vi "CycleSelection_CycleSelected_Comparison.vi"(8 "Error In":errorcluster, 10 "Board Index":i32, 11 "GEA2 Reference In":refnum<k24>) -> (0 "Error Out":errorcluster, 1 "F09D Reading":string, 2 "200A Reading":string, 3 "GEA2 Reference Out":refnum<k24>, 4 "Pass/Fail?":bool)   [LabVIEW 2016]
uses:
  Q:/Common/DLLs/GEA3/GeaCommunication.dll
  Common/DLLs/GEA3/GeaCommunication.dll
  Common/LabVIEW GEA2 Toolkit/LabVIEW_GEA2_Toolkit.lvlibp/type defs/Source_Destination.ctl
  Common/LabVIEW GEA2 Toolkit/LabVIEW_GEA2_Toolkit.lvlibp/type defs/ERD Read Data In.ctl
  Common/LabVIEW GEA2 Toolkit/LabVIEW_GEA2_Toolkit.lvlibp/type defs/Data Type.ctl
  <vilib>/regexp/Match Regular Expression.xnode
  Common/LabVIEW GEA2 Toolkit/LabVIEW_GEA2_Toolkit.lvlibp
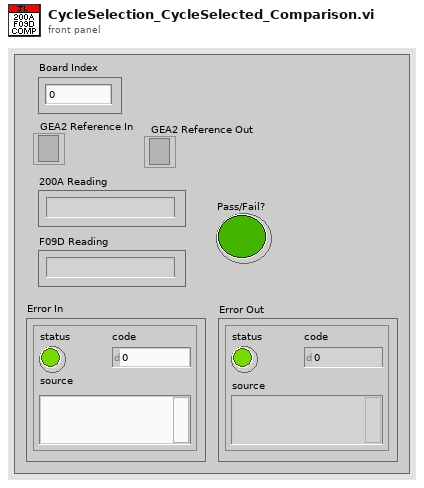
[diagram p1: front panel]
types:
  T1 = typedef "LabVIEW_GEA2_Toolkit.lvlibp/ERD Read Data In.ctl" = cluster{"ERD Number":u16, "Data Type":T2}
  T2 = typedef "LabVIEW_GEA2_Toolkit.lvlibp/Data Type.ctl" = enum16{"string", "boolean", "uint8_t", "uint16_t", "uint32_t", "uint64_t", "int8_t", "int16_t", "int32_t", "int64_t"}
  T3 = typedef "LabVIEW_GEA2_Toolkit.lvlibp/Source_Destination.ctl" = cluster{"Source":u8, "Destination":u8}
  T4 = typedef "LabVIEW_GEA2_Toolkit.lvlibp/ERD Read Data Out.ctl" = cluster{"ERD Number":u16, "Data":string}
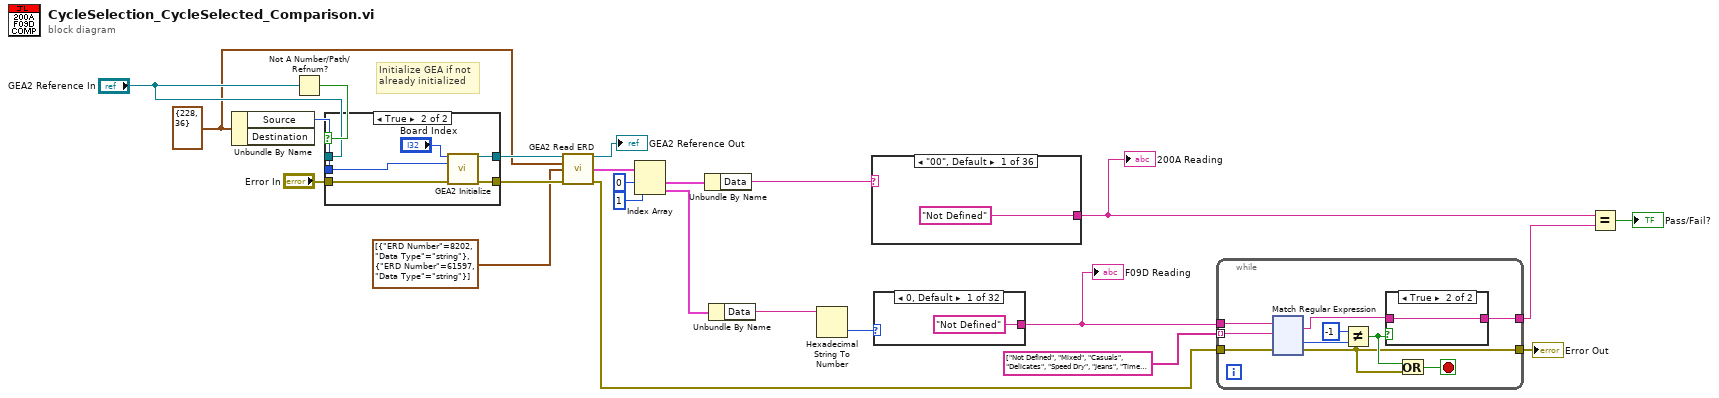
[diagram p0: block diagram]
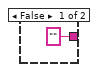
[diagram p2: hidden frame]
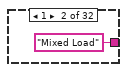
[diagram p3: hidden frame]
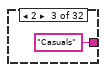
[diagram p4: hidden frame]
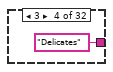
[diagram p5: hidden frame]
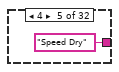
[diagram p6: hidden frame]
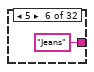
[diagram p7: hidden frame]
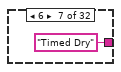
[diagram p8: hidden frame]
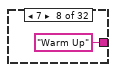
[diagram p9: hidden frame]
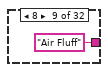
[diagram p10: hidden frame]
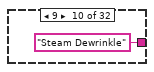
[diagram p11: hidden frame]
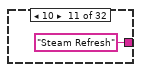
[diagram p12: hidden frame]
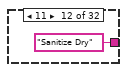
[diagram p13: hidden frame]
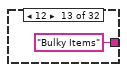
[diagram p14: hidden frame]
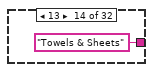
[diagram p15: hidden frame]
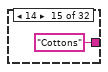
[diagram p16: hidden frame]
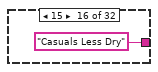
[diagram p17: hidden frame]
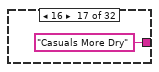
[diagram p18: hidden frame]
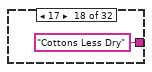
[diagram p19: hidden frame]
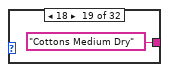
[diagram p20: hidden frame]
diagram:
  w13 = T3 {"Source"=228, "Destination"=36} ("GEA Inputs")
  # "Initialize GEA if not\nalready initialized"
  n1 = Unbundle By Name(w13) -> ("Source"=w23:u8)  [unwired: 1 out]
  n2 = Not A Number/Path/Refnum?(number/path/refnum="GEA2 Reference In") -> (NaN/Path/Refnum?=w24:bool)
  n3 = case shown="True" w24 {
    tunnel: "Error In" -> [w25 w31]
    tunnel: [w25 w30] -> w19
    tunnel: "GEA2 Reference In" -> [w26 _]
    tunnel: [w26 w29] -> w20
    tunnel: w23 -> [_ w28]
    frame False {
    }
    frame True {
      n4 = call "GEA2 Initialize.vi"("Board Index"="Board Index", "Source Address"=w28, "error in"=w31) -> ("GEA2 Reference Out"=w29:refnum<k24>, "error out"=w30:errorcluster)  [unwired: 10 in, 1 out]
    }
  }
  n5 = call "GEA2 Read ERD.vi"("GEA2 Reference In"=w20, "GEA Inputs"=w13, "Read ERD List"=T1[] [{"ERD Number"=8202, "Data Type"=enum."string"}, {"ERD Number"=61597, "Data Type"=enum."string"}], "Error In"=w19) -> ("GEA2 Reference Out"=→"GEA2 Reference Out":refnum<k24>, "ERD Data Out"=w18:T4[], "Error Out"=w6:errorcluster)  [unwired: 8 in, 1 out]
  n6 = Index Array(array=w18, index #1=0 ("index"), index #2=1 ("index")) -> (element #1=w16:T4, element #2=w10:T4)
  n7 = Unbundle By Name(w16) -> ("Data"=w15:string)
  n8 = Unbundle By Name(w10) -> ("Data"=w9:string)
  n9 = Hexadecimal String To Number(string=w9) -> (number=w14:u32)  [unwired: 2 in, 1 out]
  n10 = case shown="\"00\", Default" w15 {
    tunnel: ["Not Defined" "Basket Clean" "Drain & Spin" "Quick Rinse" "Bulky Items" "Sanitize" "Towels & Sheets" "Steam Refresh" "Normal/Mixed" "Whites" "Dark Colors" "Jeans" "Hand Wash" "Delicates" "Speed Wash" "Heavy Duty" "Allergen" "Power Clean" "Rinse & Spin" "Single Item" "Colors" "Cold Wash" "Cottons" "Easy Care" "Active Wear" "Timed Dry" "Dewrinkle" "Air Fluff" "Steam Refresh" "Steam Dewrinkle" "Speed Dry" "Mixed" "Quick Dry" "Casuals" "Warm Up" "Energy Saver"] -> w4
    frame "00", Default {
    }
    frame "01" {
    }
    frame "02" {
    }
    frame "03" {
    }
    frame "04" {
    }
    frame "05" {
    }
    frame "06" {
    }
    frame "07" {
    }
    frame "08" {
    }
    frame "09" {
    }
    frame "0A" {
    }
    frame "0B" {
    }
    frame "0C" {
    }
    frame "0D" {
    }
    frame "0E" {
    }
    frame "0F" {
    }
    frame "10" {
    }
    frame "11" {
    }
    frame "12" {
    }
    frame "13" {
    }
    frame "14" {
    }
    frame "15" {
    }
    frame "80" {
    }
    frame "81" {
    }
    frame "82" {
    }
    frame "83" {
    }
    frame "84" {
    }
    frame "85" {
    }
    frame "86" {
    }
    frame "87" {
    }
    frame "88" {
    }
    frame "89" {
    }
    frame "8A" {
    }
    frame "8B" {
    }
    frame "8C" {
    }
    frame "8D" {
    }
  }
  "200A Reading" <- w4
  n11 = case shown="0, Default" w14 {
    tunnel: ["Not Defined" ("Motor Profile") "Mixed Load" ("Motor Profile") "Casuals" ("Motor Profile") "Delicates" ("Motor Profile") "Speed Dry" ("Motor Profile") "Jeans" ("Motor Profile") "Timed Dry" ("Motor Profile") "Warm Up" ("Motor Profile") "Air Fluff" ("Motor Profile") "Steam Dewrinkle" ("Motor Profile") "Steam Refresh" ("Motor Profile") "Sanitize Dry" ("Motor Profile") "Bulky Items" ("Motor Profile") "Towels & Sheets" ("Motor Profile") "Cottons" ("Motor Profile") "Casuals Less Dry" ("Motor Profile") "Casuals More Dry" ("Motor Profile") "Cottons Less Dry" ("Motor Profile") "Cottons Medium Dry" ("Motor Profile") "Cottons More Dry" ("Motor Profile") "Delicates Less Dry" ("Motor Profile") "Delicates More Dry" ("Motor Profile") "Timed Dry 10 min" ("Motor Profile") "Timed Dry 20 min" ("Motor Profile") "Timed Dry 30 min" ("Motor Profile") "Timed Dry 40 min" ("Motor Profile") "Timed Dry 60 min" ("Motor Profile") "Timed Dry 80 min" ("Motor Profile") "Active Wear" ("Motor Profile") "Dewrinkle" ("Motor Profile") "Quick Dry" ("Motor Profile") "Energy Saver" ("Motor Profile")] -> w7
    frame 0, Default {
    }
    frame 1 {
    }
    frame 2 {
    }
    frame 3 {
    }
    frame 4 {
    }
    frame 5 {
    }
    frame 6 {
    }
    frame 7 {
    }
    frame 8 {
    }
    frame 9 {
    }
    frame 10 {
    }
    frame 11 {
    }
    frame 12 {
    }
    frame 13 {
    }
    frame 14 {
    }
    frame 15 {
    }
    frame 16 {
    }
    frame 17 {
    }
    frame 18 {
    }
    frame 19 {
    }
    frame 20 {
    }
    frame 21 {
    }
    frame 22 {
    }
    frame 23 {
    }
    frame 24 {
    }
    frame 25 {
    }
    frame 26 {
    }
    frame 27 {
    }
    frame 28 {
    }
    frame 29 {
    }
    frame 30 {
    }
    frame 31 {
    }
  }
  "F09D Reading" <- w7
  n12 = while {
    tunnel: string[] ["Not Defined", "Mixed", "Casuals", "Delicates", "Speed Dry", "Jeans", "Timed Dry", "Warm Up", "Air Fluff", "Steam Dewrinkle", "Steam Refresh", "Sanitize", "Bulky Items", "Towels & Sheets", "Active Wear", "Casuals", "Dewrinkle", "Quick Dry", "Energy Saver", "Cottons"] -> [w109] mode=indexing
    tunnel: w7 -> [w108]
    tunnel: w6 -> [w107]
    tunnel: [w102] -> w5
    tunnel: [w100] -> w3
    stop <- w101 stop-if-true
    n13 = xnode "Match Regular Expression"("input string"=w108, "regular expression"=w109, "error in"=w107) -> ("whole match"=w104:string, "offset past match"=w106:i32, "error out"=w102:errorcluster)  [unwired: 3 in, 2 out]
    n14 = Not Equal?(x=-1, y=w106) -> (x != y?=w103:bool)
    n15 = case shown="True" w103 {
      tunnel: w104 -> [_ w111]
      tunnel: ["" ("whole match") w111] -> w100
      frame False {
      }
      frame True {
      }
    }
    n16 = Or(x=w103, y=w102) -> (x .or. y?=w101:bool)
  }
  "Error Out" <- w5
  n17 = Equal?(x=w4, y=w3) -> (x = y?=→"Pass/Fail?":bool)
